vi "Main_Intlk.vi"() -> ()   [LabVIEW 2014]
uses:
  Applications/National Instruments/LabVIEW 2014/examples/Instrument IO/Serial/support/Serial - Settings.ctl
  <vilib>/Instr/_visa.llb/VISA Configure Serial Port (Instr).vi
panel:
  in  "Ring":u16(ring) items=["XXXXXXXX", "39BC6D91", "420c0e11"]
  out "Response 2":string
  in  "stop":bool
  out "Tab Control":T1(tab)
  in  "Station ID":i32
  in  "Select  VISA Resource":refnum<visa-resource-name>="ASRL2::INSTR"
  out "Resource Descriptions":string[](array[string])
  out "Response":string
  in  "Settings correct?":bool
  # "SELECT THE RESOURCE THAT\n THE READER IS ATTACHED TO:"
  # "IF CORRECT RESOURCE IS SELECTED;\nYOU SHOULD SEE A RESPONSE HERE IF\nYOU PUT DOWN AND RFID."
  # "UNIT CURRENTLY AVAILABLE..."
  # "RFID BEING CHECKED IN DATABASE..."
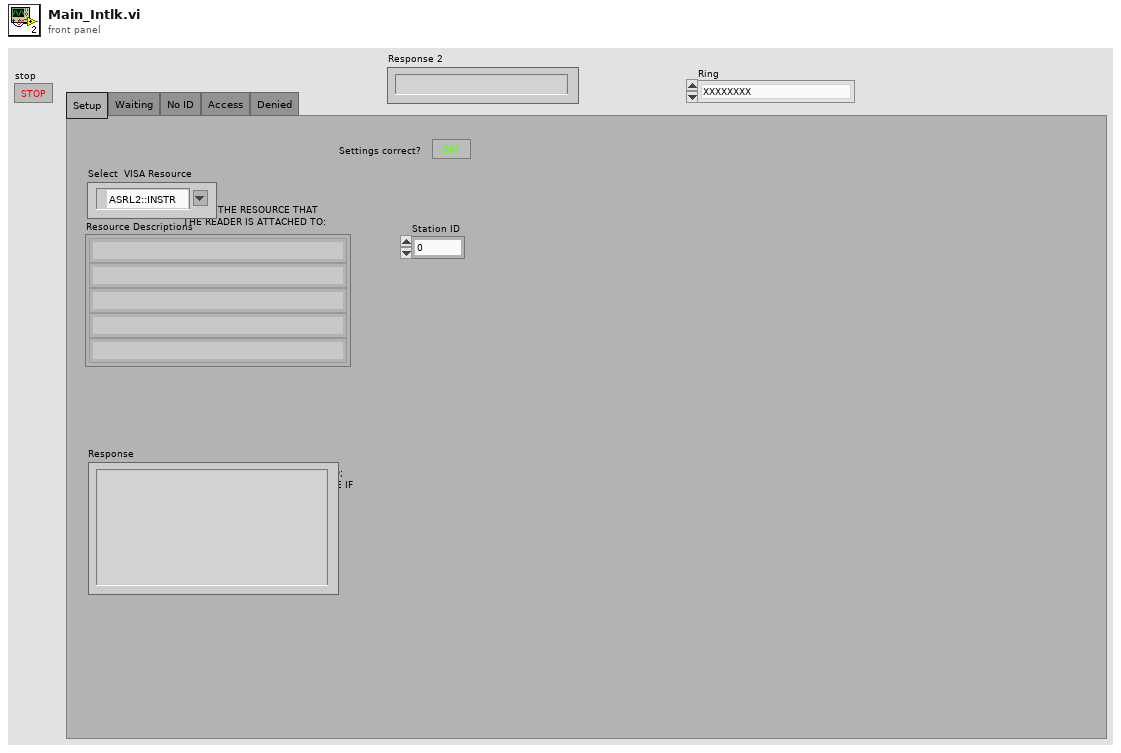
[diagram p1: front panel]
types:
  T1 = enum32{"Setup", "Waiting", "No ID", "Access", "Denied"}
  T2 = typedef "Serial - Settings.ctl" = cluster{"baud rate":u32, "data bits":u16, "parity":enum16{"None", "Odd", "Even", "Mark", "Space"}, "stop bits":u16, "flow control":u16}
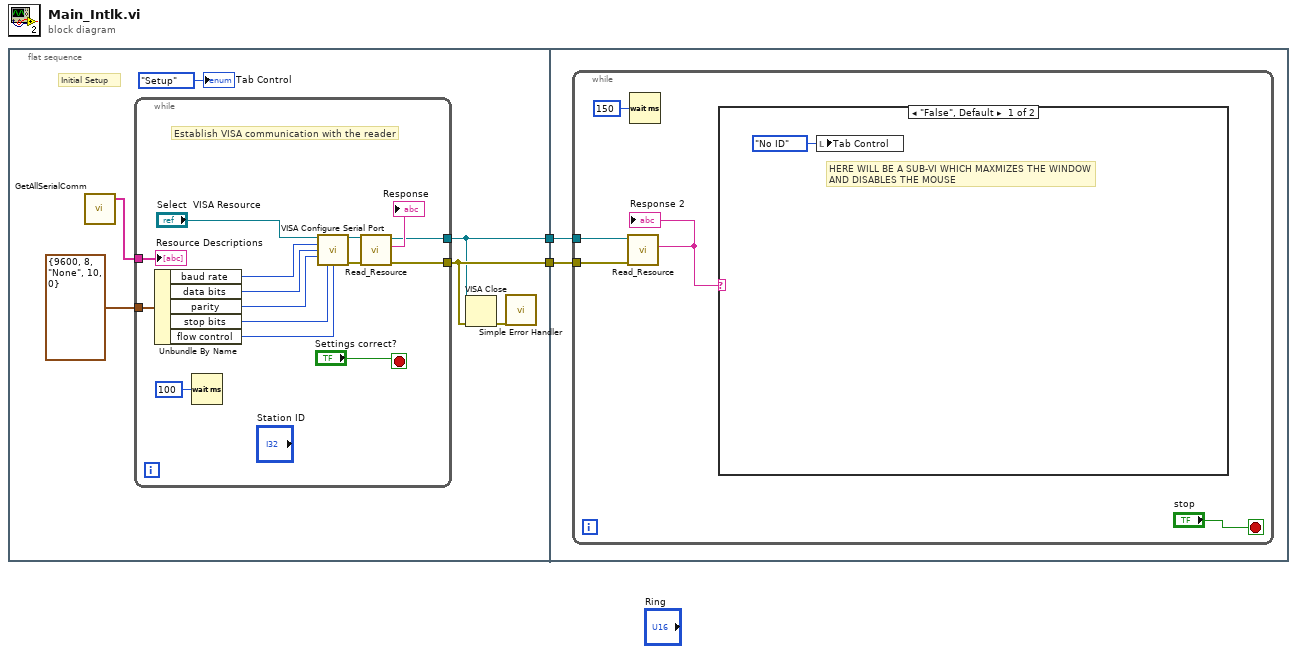
[diagram p0: block diagram]
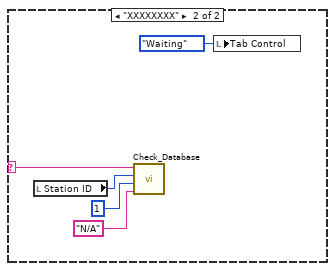
[diagram p2: hidden frame]
diagram:
  n1 = flat-sequence {
    tunnel: [w4] -> w2
    tunnel: [w3] -> w1
    tunnel: w2 -> [w25]
    tunnel: w1 -> [w24]
    frame #0 {
      # "Initial Setup"
      n2 = call "GetAllSerialComm.vi"() -> ("names"=w7:string[])  [unwired: 2 in, 2 out]
      n3 = while {
        tunnel: T2 {"baud rate"=9600, "data bits"=8, "parity"=enum."None", "stop bits"=10, "flow control"=0} ("Serial Settings") -> [w20]
        tunnel: w7 -> [w13]
        tunnel: [w11] -> w3
        tunnel: [w10] -> w4
        stop <- "Settings correct?" stop-if-true
        # "Establish VISA communication with the reader"
        n4 = Unbundle By Name(w20) -> ("baud rate"=w19:u32, "data bits"=w18:u16, "parity"=w17:enum16{"None", "Odd", "Even", "Mark", "Space"}, "stop bits"=w16:u16, "flow control"=w15:u16)
        n5 = Wait (ms)(milliseconds to wait=u32 100) -> ()  [unwired: 1 out]
        n6 = call-poly "VISA Configure Serial Port"("VISA resource name"="Select  VISA Resource", "baud rate (9600)"=w19, "data bits (8)"=w18, "parity (0:none)"=w17, "stop bits (10: 1 bit)"=w16, "flow control (0:none)"=w15) -> ("VISA resource name out"=w22:refnum<visa-resource-name>, "error out"=w23:errorcluster)  [unwired: 3 in, 5 out]
        n7 = call "Read_Resource.vi"("error in (no error)"=w23, "VISA Refnum in"=w22) -> ("error out"=w10:errorcluster, "read buffer"=→"Response":string, "VISA Refnum out"=w11:refnum<visa-resource-name>)  [unwired: 7 in]
        "Resource Descriptions" <- w13
      }
      n8 = VISA Close(VISA resource name=w3, error in (no error)=w4) -> (error out=w5:errorcluster)
      n9 = call <vilib>:"Simple Error Handler.vi"("error in (no error)"=w5) -> ()  [unwired: 1 in, 8 out]
      "Tab Control" <- T1."Setup" ("Tab Control")
    }
    frame #1 {
      n10 = while {
        tunnel: w25 -> [w30]
        tunnel: w24 -> [w29]
        stop <- "stop" stop-if-true
        n11 = call "Read_Resource.vi"("error in (no error)"=w30, "VISA Refnum in"=w29) -> ("read buffer"=w27:string)  [unwired: 7 in, 2 out]
        "Response 2" <- w27
        n12 = Wait (ms)(milliseconds to wait=u32 150) -> ()  [unwired: 1 out]
        n13 = case shown="\"False\", Default" w27 {
          selector: w27 -> [_ w32]
          frame "False", Default {
            # "HERE WILL BE A SUB-VI WHICH MAXMIZES THE WINDOW\nAND DISABLES THE MOUSE"
            n14 = local write "Tab Control"(T1."No ID" ("Tab Control")) -> ()
          }
          frame "XXXXXXXX" {
            n15 = local read "Station ID"() -> (w35:i32)
            n16 = call "Check_Database.vi"("INFO"="N/A", "REQ"=1, "STID"=w35, "RFID"=w32) -> ()  [unwired: 2 out]
            n17 = local write "Tab Control"(T1."Waiting" ("Tab Control")) -> ()
          }
        }
      }
    }
  }
